vi "Add Correction.vi"(8 "error in (no error)":errorcluster, 9 "Assembly Type":string, 10 "XYZTheta":dbl[](array[numeric]), 11 "Carrier Tray in":refnum<class "Assembly Tray.lvclass">) -> (0 "error out":errorcluster, 2 "XYZTheta Out":dbl[](array[numeric]), 3 "Carrier Tray out":refnum<class "Assembly Tray.lvclass">)   [LabVIEW 2021, in "Assembly Tray.lvclass"]
uses:
  Assembly Tray.lvclass
  C:/Users/User/Documents/Jessica_Code/Jessica_code_06052024/Gantry-CMU/UCSB-Gantry-HEP-main/Classes/Workspace/Fixture.lvclass
  Fixture.lvclass/Fixture.ctl
  Read Fixture ID.vi
  Read Position.vi
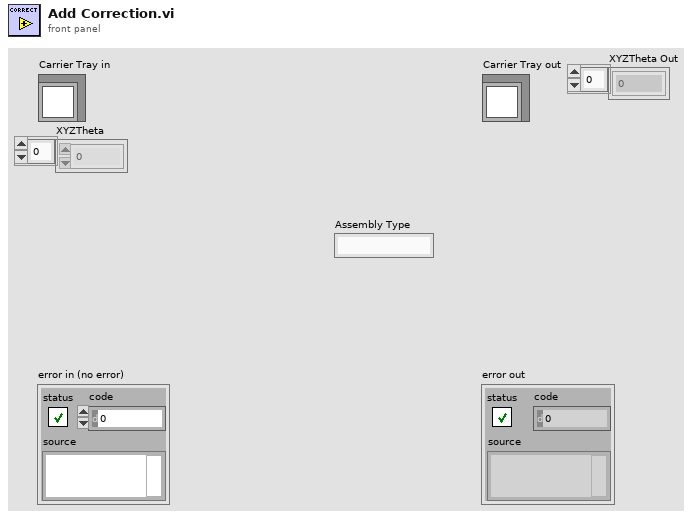
[diagram p1: front panel]
types:
  T1 = typedef "File Paths.ctl" = cluster{"Glue Pattern Folder":path, "Carrier Tray Folder":path, "Pick Up Tool Fixture Folder":path, "Components Folder":path, "Bellows Tool Offset.txt":path, "Pick Up Tool Offset.txt":path, "Dispense Tip Offset.txt":path, "Log Files":path, "Gantry Assembly Map.txt":path, "Syringe and offset map.txt":path, "Controllers Folder":path, "Local dbase config":path}
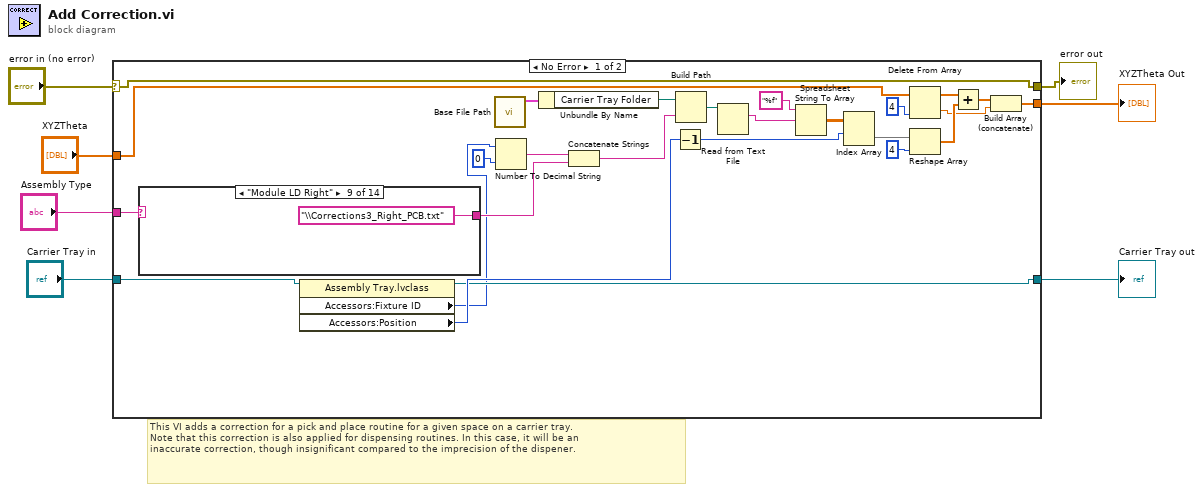
[diagram p0: block diagram]
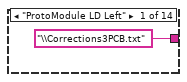
[diagram p2: hidden frame]
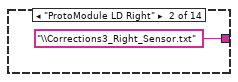
[diagram p3: hidden frame]
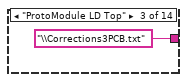
[diagram p4: hidden frame]
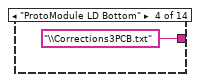
[diagram p5: hidden frame]
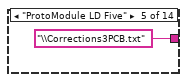
[diagram p6: hidden frame]
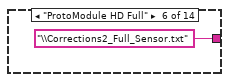
[diagram p7: hidden frame]
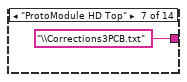
[diagram p8: hidden frame]
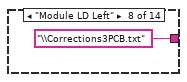
[diagram p9: hidden frame]
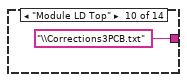
[diagram p10: hidden frame]
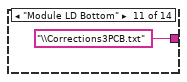
[diagram p11: hidden frame]
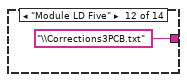
[diagram p12: hidden frame]
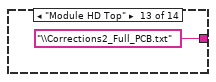
[diagram p13: hidden frame]
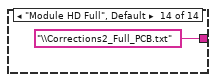
[diagram p14: hidden frame]
diagram:
  # "This VI adds a correction for a pick and place routine for a given space on a carrier tray.\nNote that this correction is also applied for dispensing routines. In this case, it will be an\ninaccurate correction, though insignificant compared to the imprecision of the dispener."
  n1 = case shown="No Error" "error in (no error)" {
    selector: "error in (no error)" -> [w33 w50]
    tunnel: [w33 w50] -> w6
    tunnel: [w16 w49] -> w4
    tunnel: "Carrier Tray in" -> [w18 w49]
    tunnel: "XYZTheta" -> [w13 w48]
    tunnel: [w8 w48] -> w2
    tunnel: "Assembly Type" -> [w14 _]
    frame No Error {
      n2 = case shown="\"Module LD Right\"" w14 {
        tunnel: ["\\Corrections3PCB.txt" ("name or relative path") "\\Corrections3_Right_Sensor.txt" ("name or relative path") "\\Corrections3PCB.txt" ("name or relative path") "\\Corrections3PCB.txt" ("name or relative path") "\\Corrections3PCB.txt" ("name or relative path") "\\Corrections2_Full_Sensor.txt" ("name or relative path") "\\Corrections3PCB.txt" ("name or relative path") "\\Corrections3PCB.txt" ("name or relative path") "\\Corrections3_Right_PCB.txt" ("name or relative path") "\\Corrections3PCB.txt" ("name or relative path") "\\Corrections3PCB.txt" ("name or relative path") "\\Corrections3PCB.txt" ("name or relative path") "\\Corrections2_Full_PCB.txt" ("name or relative path") "\\Corrections2_Full_PCB.txt" ("name or relative path")] -> w28
        frame "ProtoModule LD Left" {
        }
        frame "ProtoModule LD Right" {
        }
        frame "ProtoModule LD Top" {
        }
        frame "ProtoModule LD Bottom" {
        }
        frame "ProtoModule LD Five" {
        }
        frame "ProtoModule HD Full" {
        }
        frame "ProtoModule HD Top" {
        }
        frame "Module LD Left" {
        }
        frame "Module LD Right" {
        }
        frame "Module LD Top" {
        }
        frame "Module LD Bottom" {
        }
        frame "Module LD Five" {
        }
        frame "Module HD Top" {
        }
        frame "Module HD Full", Default {
        }
      }
      n3 = property class="Assembly Tray.lvclass"(reference=w18) -> (reference out=w16:refnum<class "Assembly Tray.lvclass">, "Accessors:Fixture ID"=w15:i32, "Accessors:Position"=w17:i32)  [unwired: 1 in, 1 out]
      n4 = call "Base File Path.vi"() -> ("Paths Out"=w32:T1)  [unwired: 11 in]
      n5 = Number To Decimal String(number=w15, width (-)=i16 0) -> (decimal integer string=w29:string)
      n6 = Unbundle By Name(w32) -> ("Carrier Tray Folder"=w31:path)
      n7 = Concatenate Strings(w29, w28) -> (w27:string)
      n8 = Decrement(x=w17) -> (x-1=w22:i32)
      n9 = Build Path(base path=w31, name or relative path=w27) -> (appended path=w26:path)
      n10 = Read from Text File(file (use dialog)=w26) -> (text=w25:string)  [unwired: 3 in, 3 out]
      n11 = Spreadsheet String To Array(format string="%f", spreadsheet string=w25) -> (array=w23:dbl[][])  [unwired: 2 in]
      n12 = Index Array(array=w23, index (row)=w22) -> (element=w20:dbl[])  [unwired: 1 in]
      n13 = Delete From Array(array=w13, index=4) -> (deleted portion=w9:dbl, array with subset deleted=w11:dbl[])  [unwired: 1 in]
      n14 = Reshape Array(w20, 4 ("dimension size")) -> (w19:dbl[])
      n15 = Add(x=w11, y=w19) -> (x+y=w10:dbl[])
      n16 = Build Array (concatenate)(w10, w9) -> (w8:dbl[])
    }
    frame Error {
    }
  }
  "error out" <- w6
  "Carrier Tray out" <- w4
  "XYZTheta Out" <- w2
